vi "Helper SubVI - Fusion Method SGL.vi"(6 "Fusion Method":cluster{"approximation":u16, "detail":u16}, 9 "Wavelet":u16, 10 "Image Pixels (Float)":dbl[][](array[numeric]), 11 "Image Pixels (Float) 2":dbl[][](array[numeric])) -> (3 "Array":sgl[][](array[numeric]))   [LabVIEW 2023]
uses:
  <vilib>/addons/Wavelet Analysis/discrete wavelet transform.llb/WA 2D Discrete Wavelet Transform.vi
  <vilib>/addons/Wavelet Analysis/discrete wavelet transform.llb/WA Inverse 2D Discrete Wavelet Transform.vi
  <vilib>/addons/_Advanced Signal Processing/NI_AdvSigProcWA.lvlib
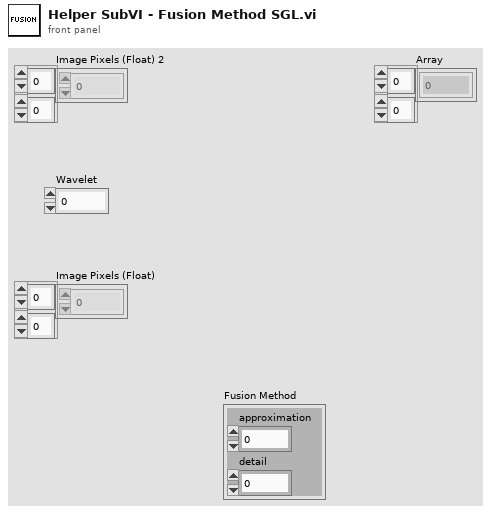
[diagram p1: front panel]
types:
  T1 = cluster{"low_low":dbl[][], "low_high":dbl[][], "high_low":dbl[][], "high_high":dbl[][]}[]
  T2 = cluster{"low_low":dbl[][], "low_high":dbl[][], "high_low":dbl[][], "high_high":dbl[][]}
  T3 = cluster{"low_low":dbl[][], "Fusion Coef":dbl[][], "Fusion Coef":dbl[][], "Fusion Coef":dbl[][]}
  T4 = cluster{"low_low":dbl[][], "Fusion Coef":dbl[][], "Fusion Coef":dbl[][], "Fusion Coef":dbl[][]}[]
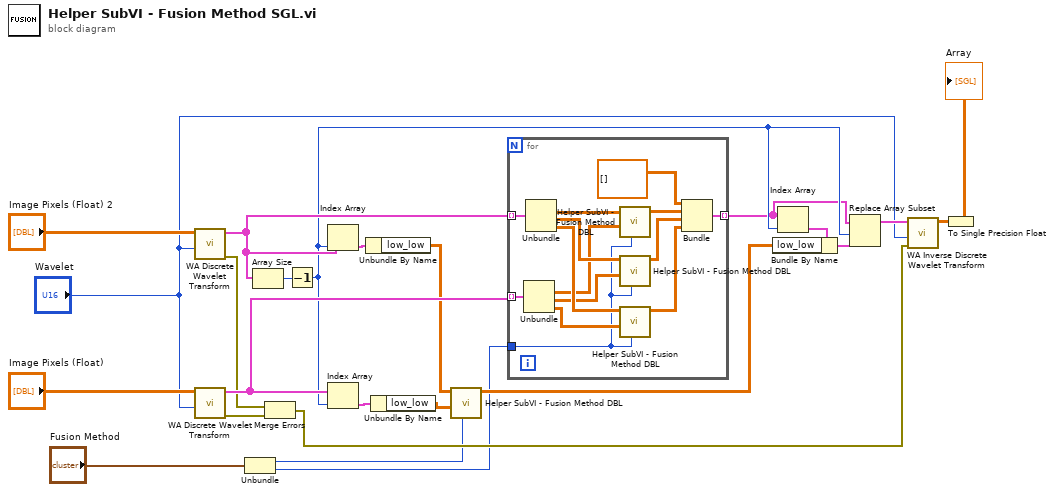
[diagram p0: block diagram]
diagram:
  n1 = call-poly <vilib>:"WA Discrete Wavelet Transform.vi"("wavelet"="Wavelet", "signal"="Image Pixels (Float) 2") -> ("error out"=w16:errorcluster, "DWT coef"=w19:T1)  [unwired: 8 in]
  n2 = call-poly <vilib>:"WA Discrete Wavelet Transform.vi"("wavelet"="Wavelet", "signal"="Image Pixels (Float)") -> ("error out"=w17:errorcluster, "DWT coef"=w20:T1)  [unwired: 8 in]
  n3 = Unbundle("Fusion Method") -> ("approximation"=w9:u16, "detail"=w10:u16)
  n4 = Array Size(array=w19) -> (size(s)=w4:i32)
  n5 = Merge Errors(w16, w17) -> (w18:errorcluster)
  n6 = Decrement(x=w4) -> (x-1=w15:i32)
  n7 = Index Array(array=w19, index=w15) -> (element=w5:T2)
  n8 = Index Array(array=w20, index=w15) -> (element=w6:T2)
  n9 = Unbundle By Name(w5) -> ("low_low"=w7:dbl[][])
  n10 = Unbundle By Name(w6) -> ("low_low"=w8:dbl[][])
  n11 = call "Helper SubVI - Fusion Method DBL.vi"("method"=w9, "Coef 2"=w8, "Coef 1"=w7) -> ("Fusion Coef"=w12:dbl[][])  [unwired: 8 in]
  n12 = for {
    tunnel: w19 -> [w38] mode=indexing
    tunnel: w20 -> [w37] mode=indexing
    tunnel: w10 -> [w30]
    tunnel: [w26] -> w13 mode=indexing
    n13 = Unbundle(w37) -> ("low_high"=w33:dbl[][], "high_low"=w32:dbl[][], "high_high"=w31:dbl[][])  [unwired: 1 out]
    n14 = Unbundle(w38) -> ("low_high"=w36:dbl[][], "high_low"=w35:dbl[][], "high_high"=w34:dbl[][])  [unwired: 1 out]
    n15 = call "Helper SubVI - Fusion Method DBL.vi"("method"=w30, "Coef 2"=w33, "Coef 1"=w36) -> ("Fusion Coef"=w29:dbl[][])  [unwired: 8 in]
    n16 = call "Helper SubVI - Fusion Method DBL.vi"("method"=w30, "Coef 2"=w32, "Coef 1"=w35) -> ("Fusion Coef"=w28:dbl[][])  [unwired: 8 in]
    n17 = call "Helper SubVI - Fusion Method DBL.vi"("method"=w30, "Coef 2"=w31, "Coef 1"=w34) -> ("Fusion Coef"=w27:dbl[][])  [unwired: 8 in]
    n18 = Bundle("low_low"=dbl[][] [], "Fusion Coef"=w29, "Fusion Coef"=w28, "Fusion Coef"=w27) -> (w26:T3)  [unwired: 1 out]
  }
  n19 = Index Array(array=w13, index=w15) -> (element=w11:T3)
  n20 = Bundle By Name(cluster=w11, "low_low"=w12) -> (w14:T3)
  n21 = Replace Array Subset(array=w13, new element=w14, index=w15) -> (w21:T4)
  n22 = call-poly <vilib>:"WA Inverse Discrete Wavelet Transform.vi"("error in (no error)"=w18, "wavelet"="Wavelet", "DWT coef"=w21) -> ("signal"=w2:dbl[][])  [unwired: 7 in, 1 out]
  n23 = To Single Precision Float(number=w2) -> (single precision float=→"Array":sgl[][])
